vi "2100_Reverse IVIO_KGD.vi"(0 "Semiconductor Module Context":T6, 1 "All_Scripts":string[][](array[string]), 2 "Master_Register_Data_Array_In":T1 {"Address" format="%.0x"}, 3 "Publishable IDs":string[](array[string])=["LowPower", "Active"], 4 "USID":T3 max=15, 5 "Error In":errorcluster, 6 "aperture time":dbl=0.001, 7 "SMU_Pins":string[](array[string])=["VSU"], 8 "Meas_Delay":dbl=0.004 format="%#_13g", 10 "Low Power_SMU_Settings":T5={"Level"=1.8, "Level Range"=6.0, "Limit"=0.001, "Limit Range"=0.001, "Sense"=1009} {"Limit" format="%#_6p"; "Limit Range" format="%#_6p"; "Sense" items=["Local"=1008, "Remote"=1009]}, 11 "HSDIO_Pins":string[](array[string])=["CLK", "SDA"], 12 "Active_SMU_Settings":T5={"Level"=1.8, "Level Range"=6.0, "Limit"=0.01, "Limit Range"=0.01, "Sense"=1009} {"Limit" format="%#_6p"; "Limit Range" format="%#_6p"; "Sense" items=["Local"=1008, "Remote"=1009]}, 13 "Script Name":string="IVIOKGD") -> (15 "Master_Register_Data_Array_Out":T1 {"Address" format="%.0x"}, 19 "Error Out":errorcluster)   [LabVIEW 2013]
uses:
  Controls/USID.ctl
  <vilib>/NI_TestStand_SemiconductorModule/NI_TestStand_Semiconductor_Module.lvlibp/PinMap/General/SemiconductorModuleContext.ctl
  <instrlib>/niDCPower/nidcpower.llb/niDCPower Sense.ctl
  Controls/Master_Reg_Data_Array.ctl
  Controls/Reg_Address_Data.ctl
  <vilib>/NI_TestStand_SemiconductorModule/NI_TestStand_Semiconductor_Module.lvlibp/PinMap/DC Power/PinsToNIDCPowerSessions.vi
  <vilib>/NI_TestStand_SemiconductorModule/NI_TestStand_Semiconductor_Module.lvlibp/PinMap/General/Publish/PublishDataDouble2D.vi
  <vilib>/NI_TestStand_SemiconductorModule/NI_TestStand_Semiconductor_Module.lvlibp/PinMap/PinQueryContext/MultiplePinMultipleSessionQueryContext/MultiplePinMultipleSessionQueryContext.lvclass
  <vilib>/NI_TestStand_SemiconductorModule/NI_TestStand_Semiconductor_Module.lvlibp
panel:
  in  "Tab Control":enum32{"Test Info", "Instrument Settings"}(tab)
  out "current measurements":dbl[][](array[numeric])
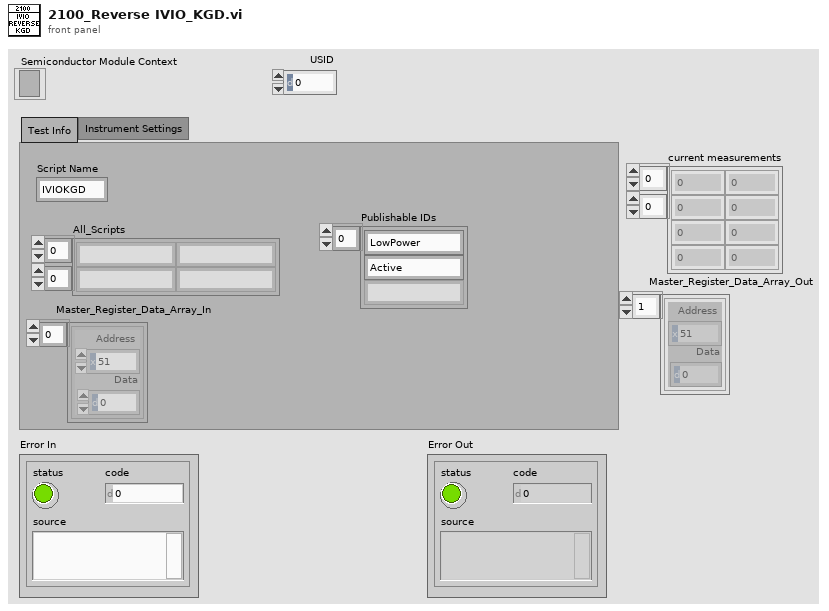
[diagram p1: front panel]
types:
  T1 = typedef "Master_Reg_Data_Array.ctl" = T2[]
  T2 = typedef "Reg_Address_Data.ctl" = cluster{"Address":u8, "Data":u8}
  T3 = typedef "USID.ctl" = u8
  T4 = typedef "niDCPower Sense.ctl" = i32
  T5 = cluster{"Level":dbl, "Level Range":dbl, "Limit":dbl, "Limit Range":dbl, "Sense":T4}
  T6 = typedef "NI_TestStand_Semiconductor_Module.lvlibp/SemiconductorModuleContext.ctl" = refnum<k7>
  T7 = typedef "Script Functions_Array.ctl" = enum16{"Reg_Write", "Bit_Write", "Delay", "Read"}[]
  T8 = enum16{"Reg_Write", "Bit_Write", "Delay", "Read"}
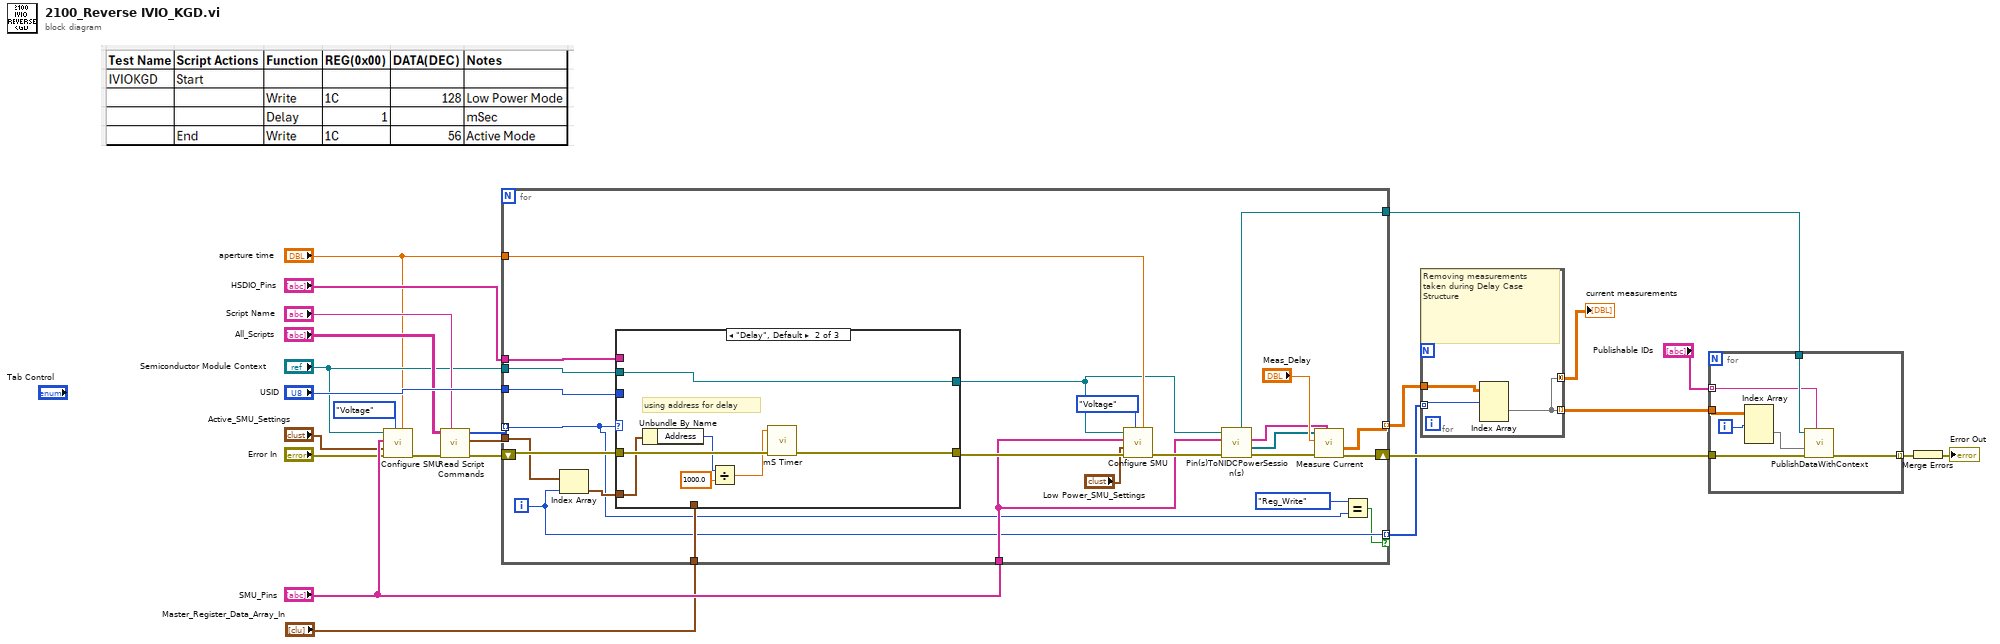
[diagram p0: block diagram]
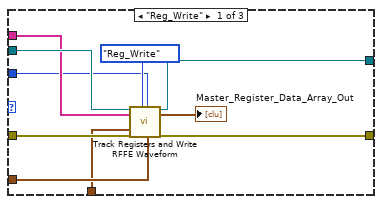
[diagram p2: hidden frame]
diagram:
  n1 = call "Configure SMU.vi"("aperture time"="aperture time", "Source Mode"=enum16{"Voltage", "Current"}."Voltage", "error in (no error)"="Error In", "Settings"="Active_SMU_Settings", "Pins"="SMU_Pins", "Semiconductor Module Context"="Semiconductor Module Context") -> ("error out"=w17:errorcluster)  [unwired: 5 in]
  n2 = call "Read Script Commands.vi"("Test Name"="Script Name", "Error In"=w17, "All_Scripts"="All_Scripts") -> ("Error Out"=w19:errorcluster, "Script_Data"=w20:T2[], "Script_Functions"=w21:T7)  [unwired: 6 in]
  n3 = for {
    tunnel: "USID" -> [w48]
    tunnel: w21 -> [w29] mode=indexing
    tunnel: w20 -> [w45]
    tunnel: "Semiconductor Module Context" -> [w47]
    tunnel: "HSDIO_Pins" -> [w46]
    tunnel: "aperture time" -> [w42]
    tunnel: "SMU_Pins" -> [w36]
    shift-right: [w31] -> w9
    shift-left: w19 -> [w49]
    tunnel: "Master_Register_Data_Array_In" -> [w33]
    tunnel: [w28] -> w2 mode=indexing if=w26
    tunnel: [w27] -> w8 mode=indexing
    tunnel: [w25] -> w5
    i -> [w28]
    n4 = Index Array(array=w45, index=w28) -> (element=w44:T2)
    n5 = case shown="\"Delay\", Default" w29 {
      tunnel: w44 -> [w53 w65 _]
      tunnel: w49 -> [w59 w66 w68]
      tunnel: w48 -> [w50 _ _]
      tunnel: w47 -> [w57 w63 w67]
      tunnel: w46 -> [w55 _ _]
      tunnel: [w58 w64 w68] -> w43
      tunnel: [w56 w63 w67] -> w37
      tunnel: w33 -> [w52 _ _]
      frame "Reg_Write" {
        n6 = call "Track Registers and Write RFFE Waveform.vi"("Semiconductor Module Context"=w57, "Pins"=w55, "Master_Register_Data_Array_In"=w52, "Error In"=w59, "Script_Functions"=enum16{"Reg_Write", "Bit_Write"}."Reg_Write", "USID"=w50, "Reg_Address_Data"=w53) -> ("Semiconductor Module Context Out"=w56:T6, "Master_Register_Data_Array_Out"=→"Master_Register_Data_Array_Out":T1, "Error Out"=w58:errorcluster)  [unwired: 10 in]
      }
      frame "Delay", Default {
        # "using address for delay"
        n7 = Unbundle By Name(w65) -> ("Address"=w61:u8)
        n8 = Divide(x=w61, y=1000.0) -> (x/y=w60:dbl)
        n9 = call "mS Timer.vi"("Error In"=w66, "Delay(S)"=w60) -> ("Error Out"=w64:errorcluster)  [unwired: 9 in]
      }
      frame "Read" {
      }
    }
    n10 = call "Configure SMU.vi"("aperture time"=w42, "Source Mode"=enum16{"Voltage", "Current"}."Voltage", "error in (no error)"=w43, "Settings"="Low Power_SMU_Settings", "Pins"=w36, "Semiconductor Module Context"=w37) -> ("error out"=w39:errorcluster)  [unwired: 5 in]
    n11 = call-poly <vilib>:"Pin(s)ToNIDCPowerSession(s).vi"("error in (no error)"=w39, "Pins"=w36, "Semiconductor Module Context"=w37) -> ("error out"=w38:errorcluster, "Instrument Sessions"=w34:refnum<k15>[], "Channel Lists"=w35:string[], "Pin Query Context"=w25:refnum<class "MultiplePinMultipleSessionQueryContext.lvclass">)  [unwired: 4 in, 1 out]
    n12 = call "Measure Current.vi"("Channel Lists"=w35, "error in (no error)"=w38, "Delay Time (s)"="Meas_Delay", "DCPower Sessions In"=w34) -> ("error out"=w31:errorcluster, "current measurements"=w27:dbl[][])  [unwired: 5 in, 1 out]
    n13 = Equal?(x=T8."Reg_Write" ("Enum"), y=w29) -> (x = y?=w26:bool)
  }
  n14 = for {
    tunnel: w8 -> [w71]
    tunnel: [w70] -> w6 mode=indexing
    tunnel: [w70] -> w7 mode=concatenating
    tunnel: w2 -> [w69] mode=indexing
    # "Removing measurements taken during Delay Case Structure"
    n15 = Index Array(array=w71, index (dim 0)=w69) -> (element=w70:dbl[][])  [unwired: 2 in]
  }
  "current measurements" <- w7
  n16 = for {
    tunnel: w9 -> [w78]
    tunnel: w6 -> [w77]
    tunnel: w5 -> [w74]
    tunnel: [w73] -> w4 mode=indexing
    tunnel: "Publishable IDs" -> [w72] mode=indexing
    i -> [w75]
    n17 = Index Array(array=w77, index (dim 0)=w75) -> (element=w76:dbl[][])  [unwired: 2 in]
    n18 = call-poly <vilib>:"PublishDataWithContext.vi"("Published Data Id"=w72, "error in (no error)"=w78, "Data In"=w76, "Pin Query Context"=w74) -> ("error out"=w73:errorcluster)  [unwired: 6 in, 1 out]
  }
  n19 = Merge Errors(w4) -> (→"Error Out":errorcluster)
